vi "ES_Packet_To_Processed_Bytes.vi"(3 "error in (no error)":errorcluster, 4 "ES Param In":T5, 5 "ES Packet In":T1) -> (0 "error out":errorcluster, 1 "Processed Bytes":u8[](array[numeric]), 2 "ES Packet Out":T1)   [LabVIEW 2017]
uses:
  Controls/Control Packets/ES_Param.ctl
  Controls/Packet/Packet.ctl
  Controls/Packet/Packet_Direction.ctl
  Controls/Packet/Packet_Type.ctl
  Controls/Packet/Packet_Priority.ctl
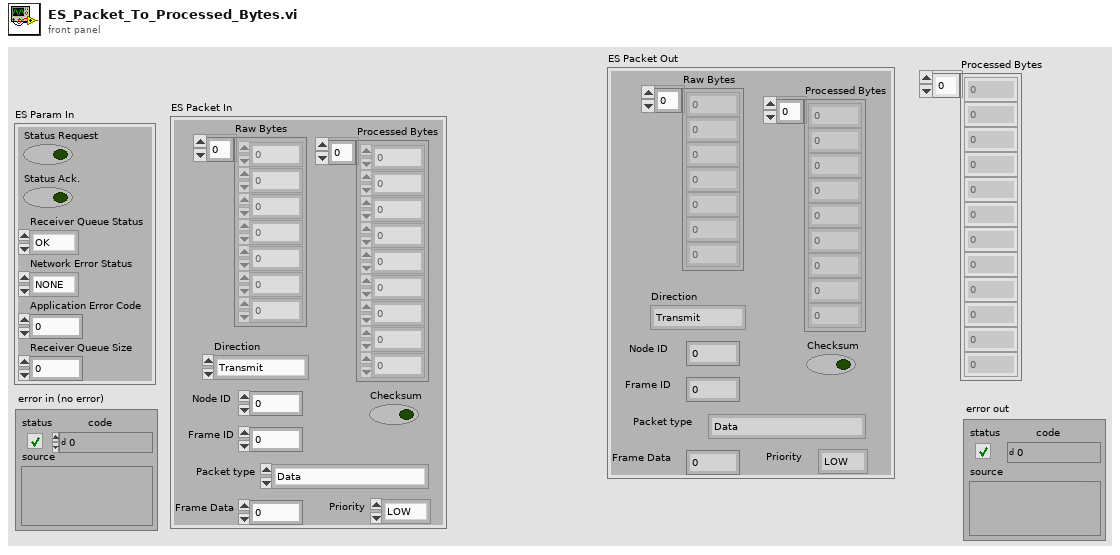
[diagram p1: front panel]
types:
  T1 = typedef "Packet.ctl" = cluster{"Raw Bytes":u8[], "Checksum":bool, "Direction":T2, "Processed Bytes":u8[], "Node ID":u8, "Packet type":T3, "Frame Data":u32, "Priority":T4, "Frame ID":u8}
  T2 = typedef "Packet_Direction.ctl" = enum16{"Transmit", "Receive", "Bidirectional"}
  T3 = typedef "Packet_Type.ctl" = enum16{"Data", "Connection Management", "Remote Request", "Error/Status"}
  T4 = typedef "Packet_Priority.ctl" = enum16{"LOW", "HIGH"}
  T5 = typedef "ES_Param.ctl" = cluster{"Status Request":bool, "Status Ack.":bool, "Receiver Queue Status":enum16{"OK", "EMPTY", "FULL"}, "Network Error Status":enum16{"NONE", "CONNECTION_ALREADY_OPEN", "CONNECTION_ALREADY_CLOSED", "INVALID_FRAME_REQUEST"}, "Application Error Code":u16, "Receiver Queue Size":i32}
  T6 = enum16{"NONE", "CONNECTION_ALREADY_OPEN", "CONNECTION_ALREADY_CLOSED", "INVALID_FRAME_REQUEST"}
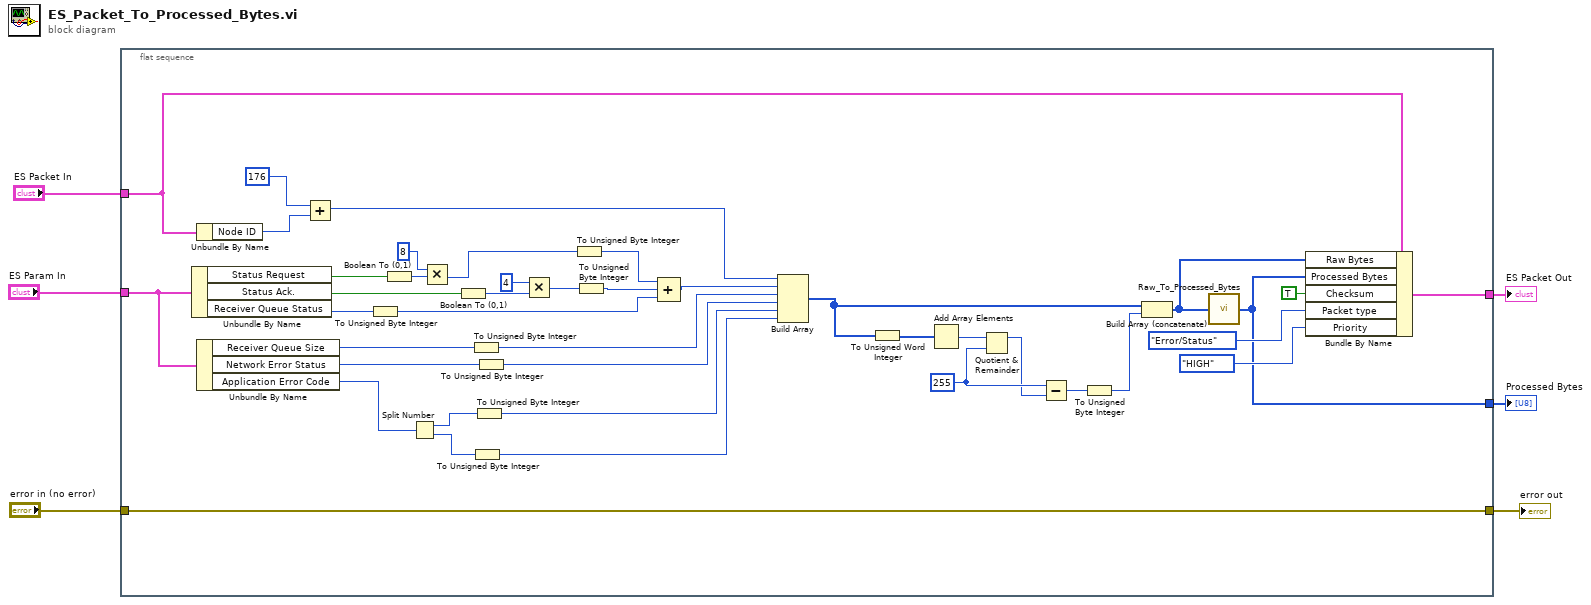
[diagram p0: block diagram]
diagram:
  n1 = flat-sequence {
    tunnel: "error in (no error)" -> [w47]
    tunnel: [w47] -> w1
    tunnel: "ES Packet In" -> [w25]
    tunnel: "ES Param In" -> [w16]
    tunnel: [w20] -> w3
    tunnel: [w19] -> w2
    frame #0 {
      w30 = u16 255 ("y")
      n2 = Unbundle By Name(w16) -> ("Status Request"=w44:bool, "Status Ack."=w43:bool, "Receiver Queue Status"=w18:enum16{"OK", "EMPTY", "FULL"})
      n3 = Unbundle By Name(w25) -> ("Node ID"=w46:u8)
      n4 = Unbundle By Name(w16) -> ("Receiver Queue Size"=w15:i32, "Network Error Status"=w14:T6, "Application Error Code"=w11:u16)
      n5 = Add(x=u8 176, y=w46) -> (x+y=w33:u8)
      n6 = To Unsigned Byte Integer(number=w18) -> (unsigned 8bit integer=w17:u8)
      n7 = Boolean To (0,1)(Boolean=w44) -> (0, 1=w42:i16)
      n8 = Split Number(x=w11) -> (hi(x)=w10:u8, lo(x)=w9:u8)
      n9 = Multiply(x=i16 8, y=w42) -> (x*y=w38:i16)
      n10 = Boolean To (0,1)(Boolean=w43) -> (0, 1=w40:i16)
      n11 = To Unsigned Byte Integer(number=w15) -> (unsigned 8bit integer=w12:u8)
      n12 = To Unsigned Byte Integer(number=w9) -> (unsigned 8bit integer=w7:u8)
      n13 = To Unsigned Byte Integer(number=w10) -> (unsigned 8bit integer=w8:u8)
      n14 = To Unsigned Byte Integer(number=w14) -> (unsigned 8bit integer=w13:u8)
      n15 = Multiply(x=i16 4, y=w40) -> (x*y=w37:i16)
      n16 = To Unsigned Byte Integer(number=w38) -> (unsigned 8bit integer=w36:u8)
      n17 = To Unsigned Byte Integer(number=w37) -> (unsigned 8bit integer=w35:u8)
      n18 = Compound Arithmetic op=ADD(w36, w35, w17) -> (w34:u8)
      n19 = Build Array(w33, w34, w12, w13, w8, w7) -> (w27:u8[])
      n20 = To Unsigned Word Integer(number=w27) -> (unsigned 16bit integer=w32:u16[])
      n21 = Add Array Elements(numeric array=w32) -> (sum=w31:u16)
      n22 = Quotient & Remainder(x=w31, y=w30) -> (x-y*floor(x/y)=w29:u16)  [unwired: 1 out]
      n23 = Subtract(x=w30, y=w29) -> (x-y=w28:u16)
      n24 = To Unsigned Byte Integer(number=w28) -> (unsigned 8bit integer=w26:u8)
      n25 = Build Array (concatenate)(w27, w26) -> (w24:u8[])
      n26 = call "Raw_To_Processed_Bytes.vi"("Raw Bytes"=w24) -> ("Processed Bytes"=w19:u8[])
      n27 = Bundle By Name(cluster=w25, "Raw Bytes"=w24, "Processed Bytes"=w19, "Checksum"=TRUE, "Packet type"=Packet_Type."Error/Status", "Priority"=Packet_Priority."HIGH") -> (w20:T1)
    }
  }
  "ES Packet Out" <- w3
  "Processed Bytes" <- w2
  "error out" <- w1
